vi "FlatToRichcif_manager_LauncherInfo.vi"(5 "OutputClusterType":T1, 11 "InputCluster":T3) -> (3 "OutputCluster":T1)   [LabVIEW 2021, in "CIF_Manager_client.lvlib"]
uses:
  CIF_Manager_client.lvlib
  cif_manager_LauncherInfo_Flat.ctl
  cif_manager_LauncherType.ctl
  cif_manager_LauncherInfo.ctl
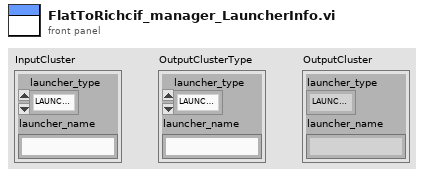
[diagram p1: front panel]
types:
  T1 = typedef "CIF_Manager_client.lvlib/cif_manager_LauncherInfo.ctl" = cluster{"launcher_type":T2, "launcher_name":string}
  T2 = typedef "CIF_Manager_client.lvlib/cif_manager_LauncherType.ctl" = enum32{"LAUNCHERTYPE_UNKNOWN", "LAUNCHERTYPE_LABVIEW"}
  T3 = typedef "CIF_Manager_client.lvlib/cif_manager_LauncherInfo_Flat.ctl" = cluster{"launcher_type":T2, "launcher_name":string}
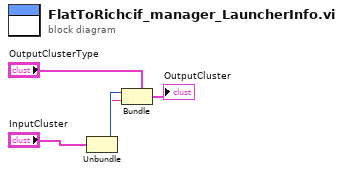
[diagram p0: block diagram]
diagram:
  n1 = Unbundle "Unbundle"("InputCluster") -> ("launcher_type"=w2:T2, "launcher_name"=w1:string)
  n2 = Bundle "Bundle"(cluster="OutputClusterType", "launcher_type"=w2, "launcher_name"=w1) -> (→"OutputCluster":T1)
